vi "Count Up U8.vi"(9 "reset value (0)":u8, 10 "reset (F)":bool, 11 "increment":bool) -> (3 "count":u8)   [LabVIEW 2013, in "I2S-TDM.lvlib"]
uses:
  I2S-TDM.lvlib
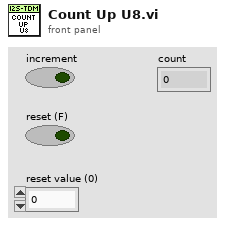
[diagram p1: front panel]
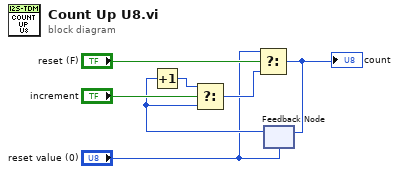
[diagram p0: block diagram]
diagram:
  n1 = feedback #1("reset value (0)") -> (w3:u8)
  n2 = Increment(x=w3) -> (x+1=w2:u8)
  n3 = Select(t=w2, s="increment", f=w3) -> (s? t:f=w6:u8)
  n4 = Select(t="reset value (0)", s="reset (F)", f=w6) -> (s? t:f=w7:u8)
  "count" <- w7
  n5 = feedback-in #1(w7) -> ()
